vi "Diesel 2.vi"() -> ()   [LabVIEW 2018]
uses:
  <vilib>/OPCUA/controls/NodeIds.ctl
  <vilib>/OPCUA/controls/NodeId.ctl
  GlobalVal.vi
  <vilib>/OPCUA/client/Multiple Read Variant.vi
  <vilib>/OPCUA/NI OPC UA Client.lvlib
panel:
  out "error out":errorcluster
  in  "DS002_Ki":dbl
  in  "DS002_Kp":dbl
  in  "DS002_tp":dbl
  in  "DS002_kP":dbl
  in  "DS002_tf":dbl
  in  "DS002_kf":dbl
  out "DS001_tf":dbl
  out "DS001_Ki":dbl
  out "DS001_tP":dbl
  out "DS001_kf":dbl
  out "DS001_kP":dbl
  out "DS001_Kp":dbl
  out "OPC Server URL":string
  out "low Level":bool
  out "DS002_f0, f Chart":cluster{dbl, dbl}(graph)
  out "DS002_P0, P Chart":cluster{dbl, dbl}(graph)
  out "Time Stamp":timestamp
  out "Pmin":dbl(slide) scale=480.0..510.0
  out "Pmax":dbl(slide) scale=480.0..510.0
  out "DS002_GasLevel":dbl(knob) scale=0.0..100.0
  in  "stop":bool
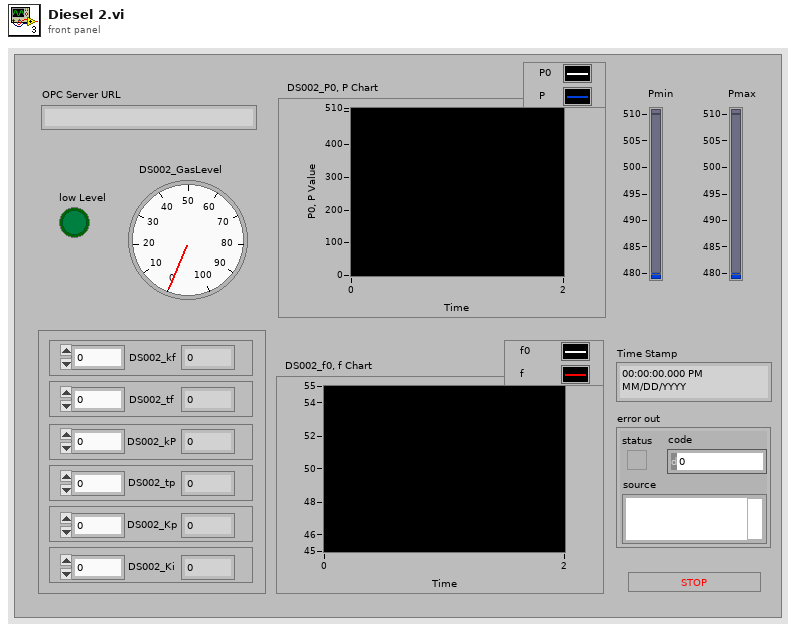
[diagram p1: front panel]
types:
  T1 = typedef "OPC UA Client Refnum.ctl" = refnum<k21>
  T2 = typedef "NodeIds.ctl" = T3[]
  T3 = typedef "NodeId.ctl" = string
  T4 = typedef "Read Variant Result.ctl" = cluster{"node ID":T3, "value ":variant, "timestamp":timestamp, "status":T5}
  T5 = typedef "OPC UA StatusCode.ctl" = u32
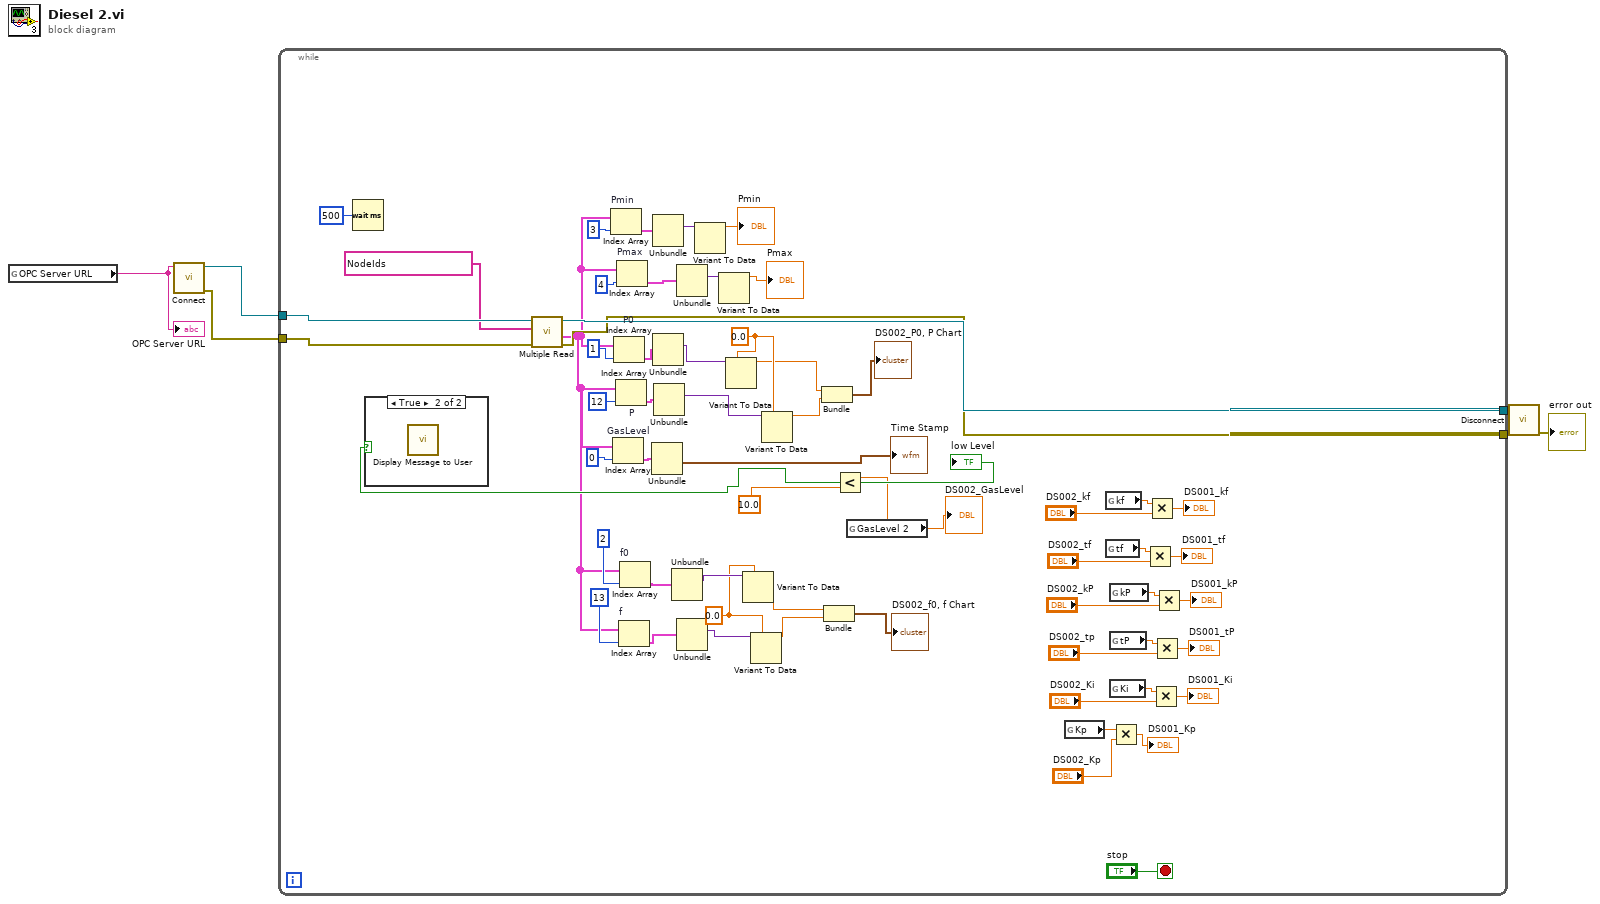
[diagram p0: block diagram]
diagram:
  n1 = global read "GlobalVal.vi" "OPC Server URL"() -> (w2:string)
  "OPC Server URL" <- w2
  n2 = call <vilib>:"Connect.vi"("server endpoint URL"=w2) -> ("error out"=w5:errorcluster, "OPC UA client refnum out"=w6:T1)  [unwired: 8 in, 1 out]
  n3 = while {
    tunnel: w6 -> [w65]
    tunnel: w5 -> [w64]
    tunnel: [w62] -> w4
    tunnel: [w61] -> w3
    stop <- "stop" stop-if-true
    w32 = 0.0
    w42 = 0.0
    n4 = Wait (ms)(milliseconds to wait=u32 500) -> ()  [unwired: 1 out]
    n5 = call-poly <vilib>:"Multiple Read.vi"("error in (no error)"=w64, "node IDs"=T2 ["ns=3;i=2", "ns=2;i=3", "ns=2;i=4", "ns=2;i=5", "ns=2;i=6", "ns=2;i=7", "ns=2;i=8", "ns=2;i=9", "ns=2;i=10", "ns=2;i=11", "ns=2;i=12", "ns=2;i=13", "ns=2;i=14", "ns=2;i=15"], "OPC UA client refnum in"=w65) -> ("error out"=w61:errorcluster, "results"=w26:T4[], "OPC UA client refnum out"=w62:T1)  [unwired: 5 in, 1 out]
    n6 = Index Array "Pmin"(array=w26, index=3) -> (element=w54:T4)
    n7 = Index Array "GasLevel"(array=w26, index=0) -> (element=w58:T4)
    n8 = Index Array "P0"(array=w26, index=1) -> (element=w56:T4)
    n9 = Index Array "P"(array=w26, index=12) -> (element=w45:T4)
    n10 = Index Array "Pmax"(array=w26, index=4) -> (element=w50:T4)
    n11 = Index Array "f"(array=w26, index=13) -> (element=w34:T4)
    n12 = Index Array "f0"(array=w26, index=2) -> (element=w37:T4)
    n13 = Unbundle(w58) -> ("timestamp"=→"Time Stamp":timestamp)  [unwired: 3 out]
    n14 = Unbundle(w54) -> ("value"=w53:variant)  [unwired: 3 out]
    n15 = Unbundle(w56) -> ("value"=w44:variant)  [unwired: 3 out]
    n16 = Unbundle(w45) -> ("value"=w43:variant)  [unwired: 3 out]
    n17 = Unbundle(w37) -> ("value"=w36:variant)  [unwired: 3 out]
    n18 = Unbundle(w50) -> ("value"=w49:variant)  [unwired: 3 out]
    n19 = Unbundle(w34) -> ("value"=w33:variant)  [unwired: 3 out]
    n20 = Variant To Data(Variant=w53) -> (data=→"Pmin":dbl)  [unwired: 2 in, 1 out]
    n21 = Variant To Data(Variant=w49) -> (data=→"Pmax":dbl)  [unwired: 2 in, 1 out]
    n22 = Variant To Data(type=w42, Variant=w44) -> (data=w39:dbl)  [unwired: 1 in, 1 out]
    n23 = Variant To Data(type=w32, Variant=w36) -> (data=w31:dbl)  [unwired: 1 in, 1 out]
    n24 = Variant To Data(type=w32, Variant=w33) -> (data=w30:dbl)  [unwired: 1 in, 1 out]
    n25 = Variant To Data(type=w42, Variant=w43) -> (data=w40:dbl)  [unwired: 1 in, 1 out]
    n26 = Bundle(w39, w40) -> (→"DS002_P0, P Chart":cluster{dbl, dbl})  [unwired: 1 in]
    n27 = Bundle(w31, w30) -> (→"DS002_f0, f Chart":cluster{dbl, dbl})  [unwired: 1 in]
    n28 = global read "GlobalVal.vi" "GasLevel 2"() -> (w25:dbl)
    "DS002_GasLevel" <- w25
    n29 = Less?(x=w25, y=10.0) -> (x < y?=w27:bool)
    "low Level" <- w27
    n30 = case shown="True" w27 {
      frame False {
      }
      frame True {
        n31 = call "Display Message to User"() -> ()  [unwired: 10 in, 2 out]
      }
    }
    n32 = global read "GlobalVal.vi" "Kp"() -> (w11:dbl)
    n33 = global read "GlobalVal.vi" "kf"() -> (w23:dbl)
    n34 = global read "GlobalVal.vi" "tf"() -> (w21:dbl)
    n35 = global read "GlobalVal.vi" "kP"() -> (w17:dbl)
    n36 = global read "GlobalVal.vi" "tP"() -> (w15:dbl)
    n37 = global read "GlobalVal.vi" "Ki"() -> (w8:dbl)
    n38 = Multiply(x=w11, y="DS002_Kp") -> (x*y=→"DS001_Kp":dbl)
    n39 = Multiply(x=w21, y="DS002_tf") -> (x*y=→"DS001_tf":dbl)
    n40 = Multiply(x=w23, y="DS002_kf") -> (x*y=→"DS001_kf":dbl)
    n41 = Multiply(x=w8, y="DS002_Ki") -> (x*y=→"DS001_Ki":dbl)
    n42 = Multiply(x=w15, y="DS002_tp") -> (x*y=→"DS001_tP":dbl)
    n43 = Multiply(x=w17, y="DS002_kP") -> (x*y=→"DS001_kP":dbl)
  }
  n44 = call <vilib>:"Disconnect.vi"("error in (no error)"=w3, "OPC UA client refnum in"=w4) -> ("error out"=→"error out":errorcluster)  [unwired: 9 in]
